vi "start forwarding device.vi"(8 "error in":errorcluster, 10 "socket 2":i32, 11 "socket 1":i32) -> (0 "error out":errorcluster)   [LabVIEW 2013, in "lvnano.lvlib"]
doc: "NN_EXPORT int nn_device (int s1, int s2);"
uses:
  lvnano.lvlib
  get last error code.vi
  get error string from code.vi
  <vilib>/Utility/error.llb/Error Cluster From Error Code.vi
  lvnanomsg.dll
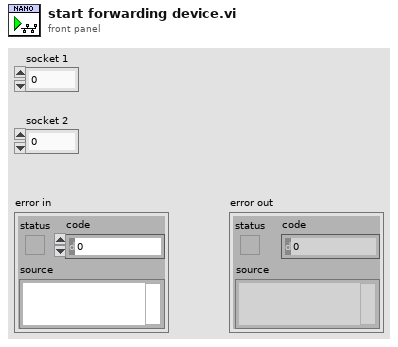
[diagram p1: front panel]
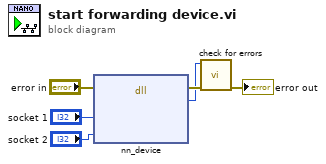
[diagram p0: block diagram]
diagram:
  n1 = dll-call lib="C:/Users/Daniel/Documents/nanomsg/lvnano/lvnanomsg.*" fn="nn_device"(error in="error in", "socket 1"="socket 1", "socket 2"="socket 2") -> (error out=w3:errorcluster, "error"=w1:i32)  [unwired: 4 in, 1 out]
  n2 = call "check for errors.vi"("error in"=w3, "function return"=w1) -> ("error out"=→"error out":errorcluster)  [unwired: 9 in]
